vi "Create UNSUBACK Packet.vi"(5 "UNSUBACK in":refnum<class "UNSUBACK.lvclass">, 8 "error in (no error)":errorcluster, 9 "Packet ID":u16 format="%04x") -> (0 "error out":errorcluster, 3 "UNSUBACK out":refnum<class "UNSUBACK.lvclass">)   [LabVIEW 2013, in "UNSUBACK.lvclass"]
uses:
  UNSUBACK.lvclass
  ControlPacket/ControlPacket.lvclass/ControlPacket.ctl
  ControlPacket/ControlPacket.lvclass
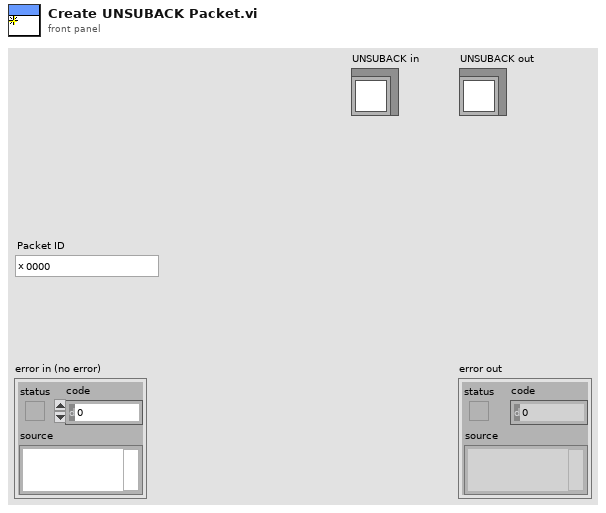
[diagram p1: front panel]
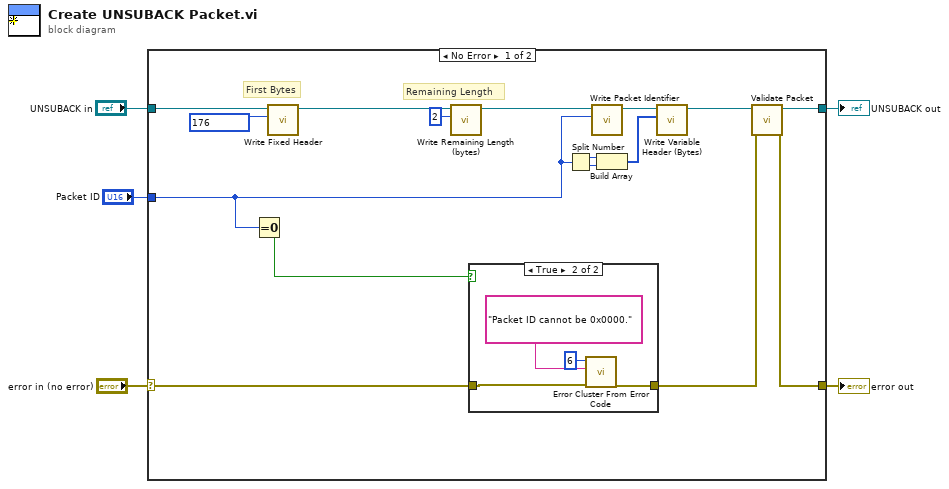
[diagram p0: block diagram]
diagram:
  n1 = case shown="No Error" "error in (no error)" {
    selector: "error in (no error)" -> [w10 w28]
    tunnel: [w7 w28] -> w2
    tunnel: [w8 w27] -> w1
    tunnel: "UNSUBACK in" -> [w21 w27]
    tunnel: "Packet ID" -> [w12 _]
    frame No Error {
      # "Remaining Length"
      # "First Bytes"
      n2 = Equal To 0?(x=w12) -> (x = 0?=w11:bool)
      n3 = call "Write Fixed Header.vi"("Fixed Header"=u8 176, "ControlPacket in"=w21) -> ("ControlPacket out"=w20:refnum<class "UNSUBACK.lvclass">)  [unwired: 9 in]
      n4 = call "Write Remaining Length (bytes).vi"("Remaining Length (bytes)"=u32 2, "ControlPacket in"=w20) -> ("ControlPacket out"=w16:refnum<class "UNSUBACK.lvclass">)  [unwired: 9 in]
      n5 = case shown="True" w11 {
        tunnel: w10 -> [w22 w25]
        tunnel: [w22 w26] -> w6
        frame False {
        }
        frame True {
          n6 = call <vilib>:"Error Cluster From Error Code.vi"("error in (no error)"=w25, "error message (\"\")"="Packet ID cannot be 0x0000.", "error code (0)"=6) -> ("error out"=w26:errorcluster)  [unwired: 6 in]
        }
      }
      n7 = Split Number(x=w12) -> (hi(x)=w19:u8, lo(x)=w18:u8)
      n8 = call "Write Packet Identifier.vi"("Packet Identifier"=w12, "ControlPacket in"=w16) -> ("ControlPacket out"=w15:refnum<class "UNSUBACK.lvclass">)  [unwired: 9 in]
      n9 = Build Array(w19, w18) -> (w17:u8[])
      n10 = call "Write Variable Header (Bytes).vi"("Variable Header (Bytes)"=w17, "ControlPacket in"=w15) -> ("ControlPacket out"=w9:refnum<class "UNSUBACK.lvclass">)  [unwired: 9 in]
      n11 = call "Validate Packet.vi"("error in (no error)"=w6, "ControlPacket in"=w9) -> ("error out"=w7:errorcluster, "ControlPacket out"=w8:refnum<class "UNSUBACK.lvclass">)  [unwired: 8 in]
    }
    frame Error {
    }
  }
  "error out" <- w2
  "UNSUBACK out" <- w1
